vi "Test Some Other Test Method.vi"(8 "error in (no error)":errorcluster, 11 "Global Fixture Test Double in":refnum<class "Global Fixture Test Double.lvclass">) -> (0 "error out":errorcluster, 3 "Global Fixture Test Double out":refnum<class "Global Fixture Test Double.lvclass">)   [LabVIEW 2020, in "Global Fixture Test Double.lvclass"]
uses:
  Global Fixture Test Double.lvclass
  C:/Program Files (x86)/National Instruments/LabVIEW 2020/vi.lib/Astemes/LUnit/Test Case.lvclass
  <vilib>/Astemes/LUnit/Test Case.lvclass/Test Case.ctl
  <vilib>/Astemes/LUnit/Append Fail Result.vi
  <vilib>/Astemes/LUnit/Append Pass Result.vi
  Global Fixture Test Double.lvclass/Global Fixture Test Double.ctl
  <vilib>/Astemes/LUnit/Test Case.lvclass
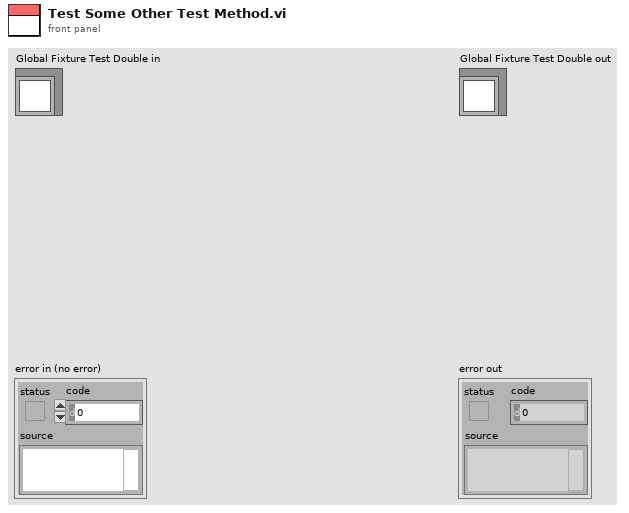
[diagram p1: front panel]
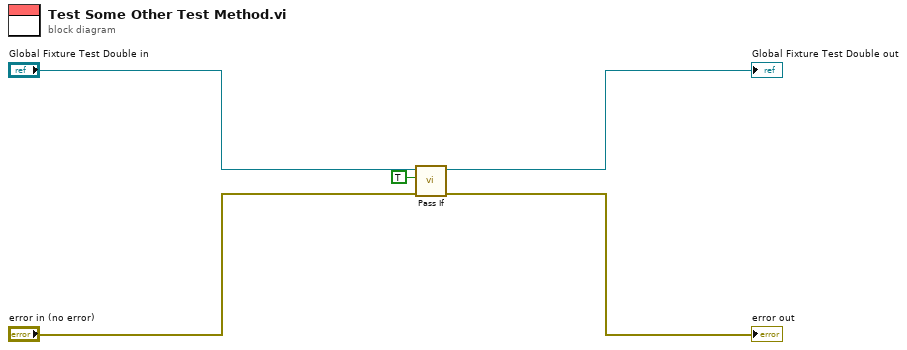
[diagram p0: block diagram]
diagram:
  n1 = call <vilib>:"Pass If.vi"("error in (no error)"="error in (no error)", "Pass?"=TRUE, "LUnit Test Case In"="Global Fixture Test Double in") -> ("error out"=→"error out":errorcluster, "LUnit Test Case Out"=→"Global Fixture Test Double out":refnum<class "Global Fixture Test Double.lvclass">)  [unwired: 7 in]
